vi "17.DMA-FIFO (Host).vi"() -> ()   [LabVIEW 2019]
uses:
  <vilib>/rvi/interface/nirviOpenFPGA/nirviOpenFPGA.xnode
  <vilib>/rvi/interface/nirviMethod/nirviMethod.xnode
  <vilib>/FPGAPlugInAG/ELVIS III/niLvFpga_ConfigureFifo_ELVIS III.vi
  <vilib>/rvi/errors/niLvFpgaMergeErrorWithErrorCode.vi
  <vilib>/FPGAPlugInAG/ELVIS III/niLvFpga_ReadFifo_ELVIS III.vi
  <vilib>/rvi/interface/nirviReadWriteControl/nirviReadWriteControl.xnode
  NiFpgaLv.dll
  <vilib>/Utility/error.llb/Error Cluster From Error Code.vi
  <vilib>/rvi/errors/niLvFpgaAdjustHostInterfaceError.vi
  <vilib>/rvi/interface/nirviCloseFPGA/nirviCloseFPGA.xnode
  <vilib>/FPGAPlugInAG/ELVIS III/niLvFpga_Close_ELVIS III.vi
panel:
  out "error out":errorcluster
  out "Overflow Count":u32
  in  "stop":bool
  out "Flushed Data":dbl[](array[numeric])
  out "Data":dbl[](graph)
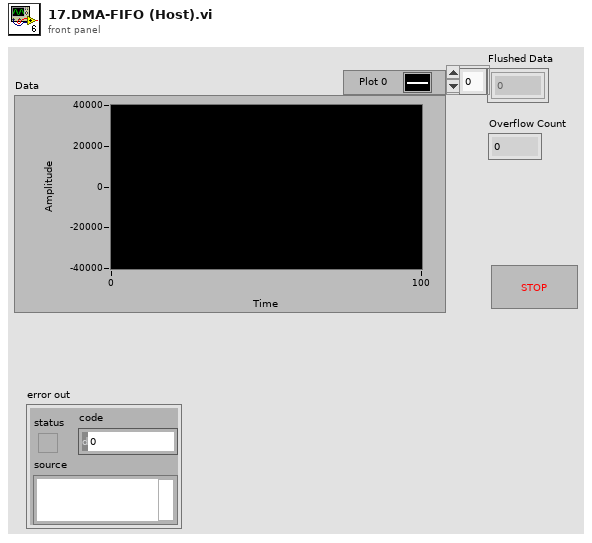
[diagram p1: front panel]
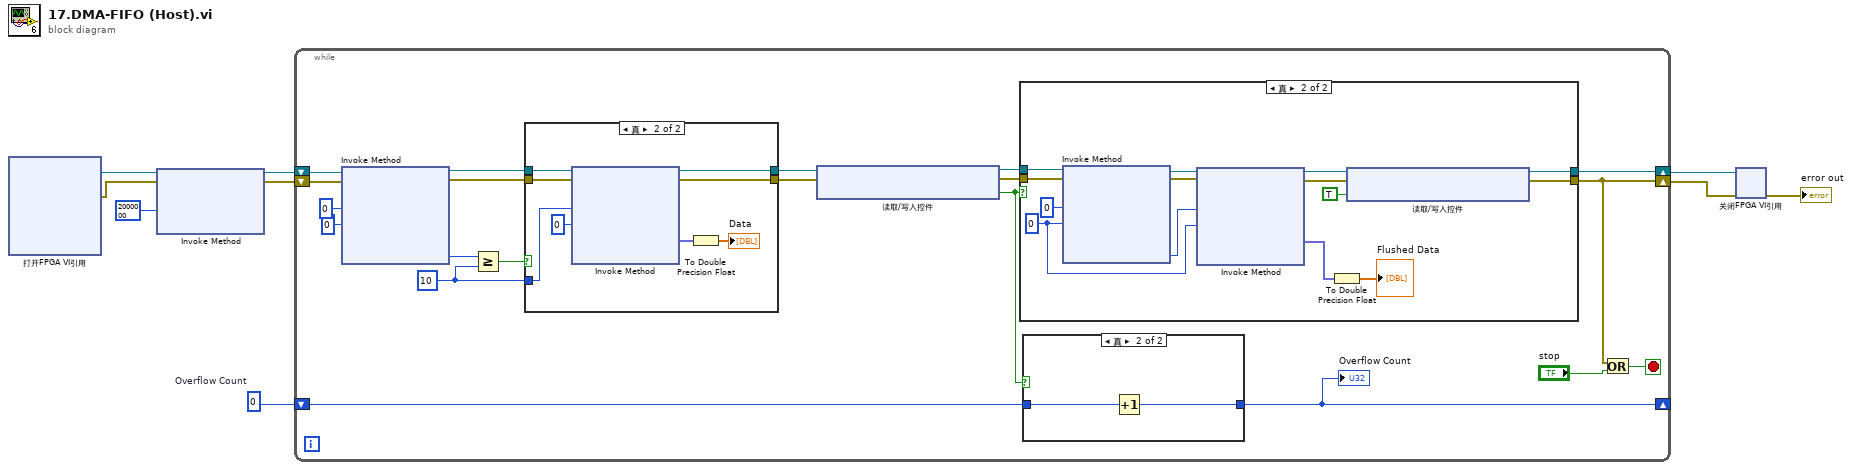
[diagram p0: block diagram]
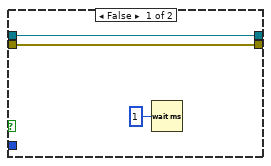
[diagram p4: hidden frame]
diagram:
  w4 = u32 0  # Overflow Count
  n1 = xnode "打开FPGA VI引用"() -> ("FPGA VI引用输出"=w9:refnum<k20>, "错误输出"=w8:errorcluster)  [unwired: 2 in]
  n2 = xnode "Invoke Method"("FPGA VI引用输入"=w9, "错误输入"=w8, "请求的深度"=u32 2000000 ("Depth")) -> ("FPGA VI引用输出"=w6:refnum<k20>, "错误输出"=w5:errorcluster)  [unwired: 1 out]
  n3 = while {
    shift-right: [w16] -> w3
    shift-left: w6 -> [w28]
    shift-right: [w12] -> w2
    shift-left: w5 -> [w29]
    shift-right: [w10] -> _
    shift-left: w4 -> [w15]
    stop <- w13 stop-if-true
    w23 = u32 10 ("y")
    n4 = xnode "Invoke Method"("FPGA VI引用输入"=w28, "错误输入"=w29, "元素数量"=u32 0, "超时(ms)"=0) -> ("FPGA VI引用输出"=w21:refnum<k20>, "错误输出"=w22:errorcluster, "剩余元素"=w25:u32)  [unwired: 1 out]
    n5 = Greater Or Equal?(x=w25, y=w23) -> (x >= y?=w24:bool)
    n6 = case shown="真" w24 {
      tunnel: w23 -> [_ w57]
      tunnel: w22 -> [w51 w59]
      tunnel: w21 -> [w50 w58]
      tunnel: [w51 w53] -> w20
      tunnel: [w50 w52] -> w19
      frame False {
        n7 = Wait (ms)(milliseconds to wait=u32 1 ("等待时间（毫秒）")) -> ()  [unwired: 1 out]
      }
      frame True {
        n8 = xnode "Invoke Method"("FPGA VI引用输入"=w58, "错误输入"=w59, "元素数量"=w57, "超时(ms)"=0) -> ("FPGA VI引用输出"=w52:refnum<k20>, "错误输出"=w53:errorcluster, "数据"=w55:fxp<+/-,24,5>[])  [unwired: 1 out]
        n9 = To Double Precision Float(number=w55) -> (double precision float=→"Data":dbl[])
      }
    }
    n10 = xnode "读取/写入控件"("FPGA VI引用输入"=w19, "错误输入"=w20) -> ("FPGA VI引用输出"=w17:refnum<k20>, "错误输出"=w18:errorcluster, "Overflow?"=w14:bool)
    n11 = case shown="真" w14 {
      tunnel: w18 -> [w34 w48]
      tunnel: w17 -> [w33 w47]
      tunnel: [w34 w36] -> w12
      tunnel: [w33 w35] -> w16
      frame False {
      }
      frame True {
        w42 = 0 ("超时(ms)")
        n12 = xnode "Invoke Method"("FPGA VI引用输入"=w47, "错误输入"=w48, "元素数量"=u32 0, "超时(ms)"=w42) -> ("FPGA VI引用输出"=w44:refnum<k20>, "错误输出"=w45:errorcluster, "剩余元素"=w43:u32)  [unwired: 1 out]
        n13 = xnode "Invoke Method"("FPGA VI引用输入"=w44, "错误输入"=w45, "元素数量"=w43, "超时(ms)"=w42) -> ("FPGA VI引用输出"=w38:refnum<k20>, "错误输出"=w39:errorcluster, "数据"=w41:fxp<+/-,24,5>[])  [unwired: 1 out]
        n14 = To Double Precision Float(number=w41) -> (double precision float=→"Flushed Data":dbl[])
        n15 = xnode "读取/写入控件"("FPGA VI引用输入"=w38, "错误输入"=w39, "DMA Cleared?"=TRUE) -> ("FPGA VI引用输出"=w35:refnum<k20>, "错误输出"=w36:errorcluster)
      }
    }
    n16 = case shown="真" w14 {
      tunnel: w15 -> [w30 w32]
      tunnel: [w30 w31] -> w10
      frame False {
      }
      frame True {
        n17 = Increment(x=w32) -> (x+1=w31:u32)
      }
    }
    "Overflow Count" <- w10
    n18 = Or(x=w12, y="stop") -> (x .or. y?=w13:bool)
  }
  n19 = xnode "关闭FPGA VI引用"("FPGA VI引用输入"=w3, "错误输入"=w2) -> ("错误输出"=→"error out":errorcluster)
